vi "Device VI 1.4.vi"() -> ()   [LabVIEW 2017]
uses:
  <vilib>/Utility/error.llb/DialogType.ctl
  <vilib>/DAQmx/read.llb/DAQmx Read (Analog 1D Wfm NChan NSamp).vi
  <vilib>/DAQmx/create/channels.llb/DAQmx Create Channel (AI-Force-Bridge-Two-Point-Linear).vi
  <vilib>/DAQmx/configure/timing.llb/DAQmx Timing (Sample Clock).vi
  <vilib>/DAQmx/configure/trigger.llb/DAQmx Start Trigger (Digital Edge).vi
  <vilib>/DAQmx/configure/trigger.llb/DAQmx Start Trigger (Analog Edge).vi
  <vilib>/DAQmx/miscellaneous.llb/DAQmx Fill In Error Info.vi
  <resource>/objmgr/daqmx.rc
panel:
  in  "Pause":bool
  in  "Start":bool
  in  "Stop 3":bool
  in  "Spreadsheet Location":path=path "C:/Users/Julio/Desktop/Device Data/Test 2.xlsx" caption="Filename"
  in  "Units (Force)":i32(ring)=15875 items=["Newtons"=15875, "Pounds"=15876, "kgf"=15877, "From Custom Scale"=10065]
  in  "Physical Channel":tag="cDAQ2Mod1/ai0:1"
  in  "Sample Rate (Hz)":dbl=100.0
  in  "Samples per Loop":i32=100
  in  "scaling information":T1={"first electrical value"=0.0, "second electrical value"=2.0, "electrical units"=15897, "first physical value"=0.0, "second physical value"=100.0, "physical units"=15876} {"physical units" items=["Newtons"=15875, "Pounds"=15876, "kgf"=15877]; "electrical units" items=["Volts/Volt"=15896, "mVolts/Volt"=15897]}
  in  "Maximum Force":dbl=100.0
  in  "Minimum Force":dbl=-100.0
  in  "Trigger Type":T2(tab)
  in  "Digital Start Trigger Edge":i32(ring)=10280 caption="Edge" items=["Rising"=10280, "Falling"=10171]
  in  "Digital Start Trigger Source":tag="OnboardClock" caption="Source"
  in  "Digital Pause Trigger Pause When":i32(ring)=10192 caption="Pause When" items=["High"=10192, "Low"=10214]
  in  "Digital Pause Trigger Source":tag="/Dev1/PFI0" caption="Source"
  in  "Analog Start Trigger Level":dbl caption="Level" format="%0.2f"
  in  "Analog Start Trigger Hysteresis":dbl caption="Hysteresis" format="%.2f"
  in  "Analog Start Trigger Slope":i32(ring)=10280 caption="Slope" items=["Rising"=10280, "Falling"=10171]
  in  "Analog Start Trigger Source":string="APFI0" caption="Source"
  in  "Analog Pause Trigger Source":string="APFI0" caption="Source"
  in  "Analog Pause Trigger Pause When":i32(ring)=10093 caption="Pause When" items=["Above Level"=10093, "Below Level"=10107]
  in  "Analog Pause Trigger Level":dbl caption="Level" format="%.2f"
  in  "Bridge Information":T3={"Bridge Configuration"=10182, "Excitation Source"=10200, "Excitation Value"=2.5, "Nominal Resistance"=350.0} {"Excitation Source" items=["Internal"=10200, "External"=10167, "None"=10230]; "Bridge Configuration" items=["Full Bridge"=10182, "Half Bridge"=10187, "Quarter Bridge"=10270, "No Bridge"=10228]}
  out "Waveform Chart":waveform(dbl)[](graph)=[{"t0"=timestamp(3612864703.636625 s since 1904-01-01), "dt"=0.01, "Y"=[-0.0008285458908220164, -0.0008285458908220164, -0.0008285458908220164, -0.0008285458908220164, -0.0008285458908220164, -0.0008285458908220164, -0.0008285458908220164, -0.0008285458908220164, -0.0008285458908220164, -0.0008285458908220164, -0.0008285458908220164, -0.0008285458908220164, -0.0008285458908220164, -0.0008285458908220164, -0.0008285458908220164, -0.0008285458908220164, -0.0008285458908220164, -0.0008285458908220164, -0.0008285458908220164, -0.0008285458908220164, -0.0008285458908220164, -0.0008285458908220164, -0.0008285458908220164, -0.0008285458908220164, -0.0008285458908220164, -0.0008285458908220164, -0.0008285458908220164, -0.0008285458908220164, -0.0008285458908220164, -0.0008285458908220164, -0.0008285458908220164, -0.0008285458908220164, -0.0008285458908220164, -0.0008285458908220164, -0.0008285458908220164, -0.0008285458908220164, -0.0008285458908220164, -0.0008285458908220164, -0.0008285458908220164, -0.0008285458908220164, -0.0008285458908220164, -0.0008285458908220164, -0.0008285458908220164, -0.0008285458908220164, -0.0008285458908220164, -0.0008285458908220164, -0.0008285458908220164, -0.0008285458908220164, -0.0008285458908220164, -0.0008285458908220164, -0.0008285458908220164, -0.0008285458908220164, -0.0008285458908220164, -0.0008285458908220164, -0.0008285458908220164, -0.0008285458908220164, -0.0008285458908220164, -0.0008285458908220164, -0.0008285458908220164, -0.0008285458908220164, -0.0008285458908220164, -0.0008285458908220164, -0.0008285458908220164, -0.0008285458908220164, -0.0008285458908220164, -0.0008285458908220164, -0.0008285458908220164, -0.0008285458908220164, -0.0008285458908220164, -0.0008285458908220164, -0.0008285458908220164, -0.0008285458908220164, -0.0008285458908220164, -0.0008285458908220164, -0.0008285458908220164, -0.0008285458908220164, -0.0008285458908220164, -0.0008285458908220164, -0.0008285458908220164, -0.0008285458908220164, -0.0008285458908220164, -0.0008285458908220164, -0.0008285458908220164, -0.0008285458908220164, -0.0008285458908220164, -0.0008285458908220164, -0.0008285458908220164, -0.0008285458908220164, -0.0008285458908220164, -0.0008285458908220164, -0.0008285458908220164, -0.0008285458908220164, -0.0008285458908220164, -0.0008285458908220164, -0.0008285458908220164, -0.0008285458908220164, -0.0008285458908220164, -0.0008285458908220164, -0.0008285458908220164, -0.0008285458908220164], "attributes"=variant("NI_ChannelName"=variant(string "cDAQ2Mod1/ai0"), "NI_UnitDescription"=variant(string "Newtons"))}, {"t0"=timestamp(3612864703.636625 s since 1904-01-01), "dt"=0.01, "Y"=[0.006835503599282382, 0.006835503599282382, 0.006835503599282382, 0.006835503599282382, 0.006835503599282382, 0.006835503599282382, 0.006835503599282382, 0.006835503599282382, 0.006835503599282382, 0.006835503599282382, 0.006835503599282382, 0.006835503599282382, 0.006835503599282382, 0.006835503599282382, 0.006835503599282382, 0.006835503599282382, 0.006835503599282382, 0.006835503599282382, 0.006835503599282382, 0.006835503599282382, 0.006835503599282382, 0.006835503599282382, 0.006835503599282382, 0.006835503599282382, 0.006835503599282382, 0.006835503599282382, 0.006835503599282382, 0.006835503599282382, 0.006835503599282382, 0.006835503599282382, 0.006835503599282382, 0.006835503599282382, 0.006835503599282382, 0.006835503599282382, 0.006835503599282382, 0.006835503599282382, 0.006835503599282382, 0.006835503599282382, 0.006835503599282382, 0.006835503599282382, 0.006835503599282382, 0.006835503599282382, 0.006835503599282382, 0.006835503599282382, 0.006835503599282382, 0.006835503599282382, 0.006835503599282382, 0.006835503599282382, 0.006835503599282382, 0.006835503599282382, 0.008906868326337657, 0.008906868326337657, 0.008906868326337657, 0.008906868326337657, 0.008906868326337657, 0.008906868326337657, 0.008906868326337657, 0.008906868326337657, 0.008906868326337657, 0.008906868326337657, 0.008906868326337657, 0.008906868326337657, 0.008906868326337657, 0.008906868326337657, 0.008906868326337657, 0.008906868326337657, 0.008906868326337657, 0.008906868326337657, 0.008906868326337657, 0.008906868326337657, 0.008906868326337657, 0.008906868326337657, 0.008906868326337657, 0.008906868326337657, 0.008906868326337657, 0.008906868326337657, 0.008906868326337657, 0.008906868326337657, 0.008906868326337657, 0.008906868326337657, 0.008906868326337657, 0.008906868326337657, 0.008906868326337657, 0.008906868326337657, 0.008906868326337657, 0.008906868326337657, 0.008906868326337657, 0.008906868326337657, 0.008906868326337657, 0.008906868326337657, 0.008906868326337657, 0.008906868326337657, 0.008906868326337657, 0.008906868326337657, 0.008906868326337657, 0.008906868326337657, 0.008906868326337657, 0.008906868326337657, 0.008906868326337657, 0.008906868326337657], "attributes"=variant("NI_ChannelName"=variant(string "cDAQ2Mod1/ai1"), "NI_UnitDescription"=variant(string "Newtons"))}]
  # "Settings"
  # "This trigger type is not supported in continuous sample timing. \n\nRefer to your device documentation for more information on which triggers are supported."
  # "This trigger type is not supported in continuous sample timing. \n\nRefer to your device documentation for more information on which triggers are supported."
  # "Data"
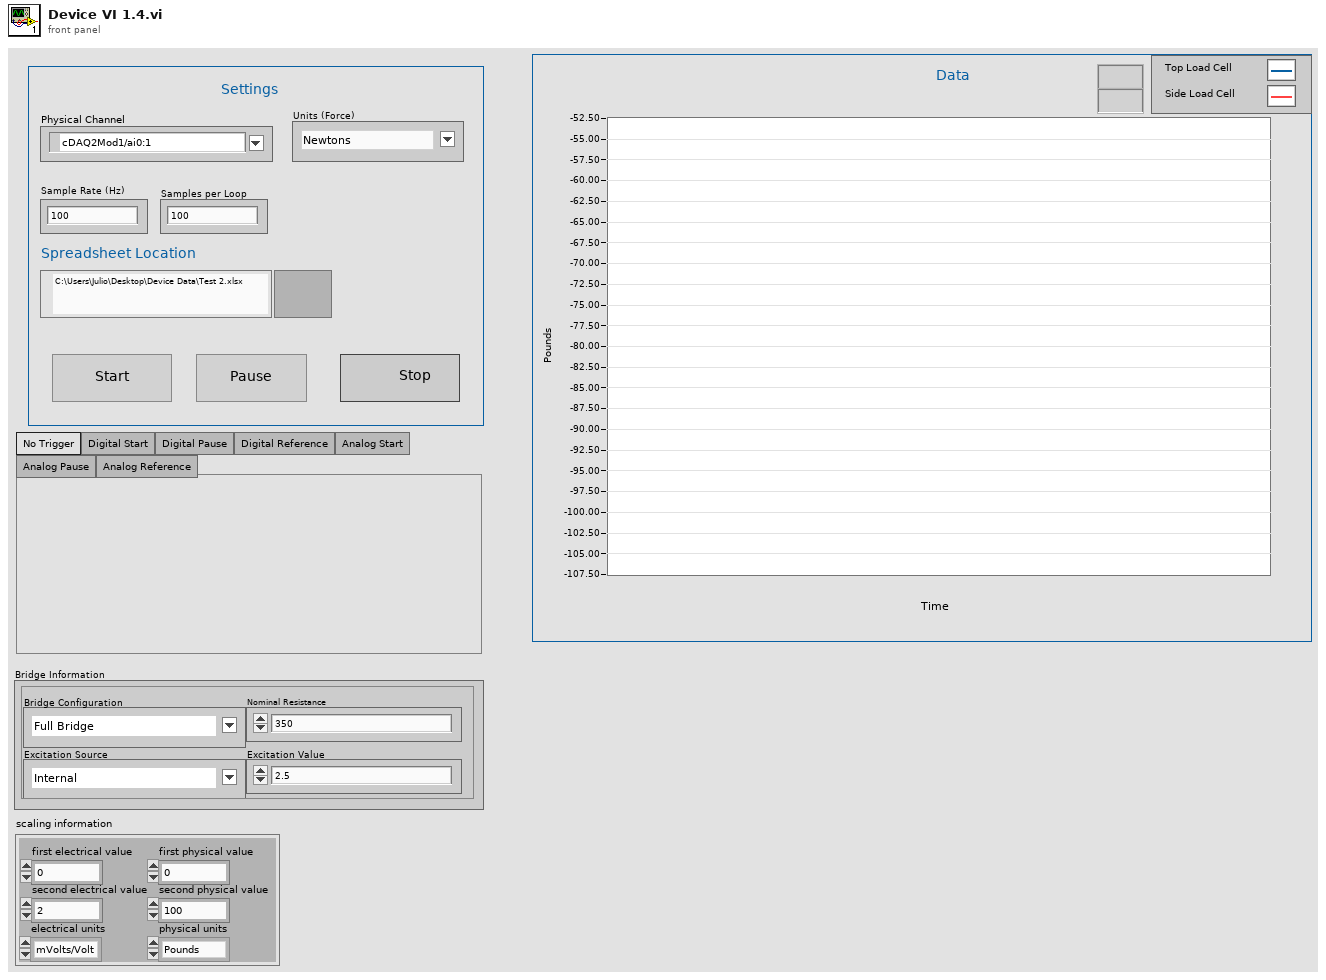
[diagram p1: front panel]
types:
  T1 = cluster{"first electrical value":dbl, "second electrical value":dbl, "electrical units":i32, "first physical value":dbl, "second physical value":dbl, "physical units":i32}
  T2 = enum32{"No Trigger", "Digital Start", "Digital Pause", "Digital Reference", "Analog Start", "Analog Pause", "Analog Reference"}
  T3 = cluster{"Bridge Configuration":i32, "Excitation Source":i32, "Excitation Value":dbl, "Nominal Resistance":dbl}
  T4 = typedef "DialogType.ctl" = u16
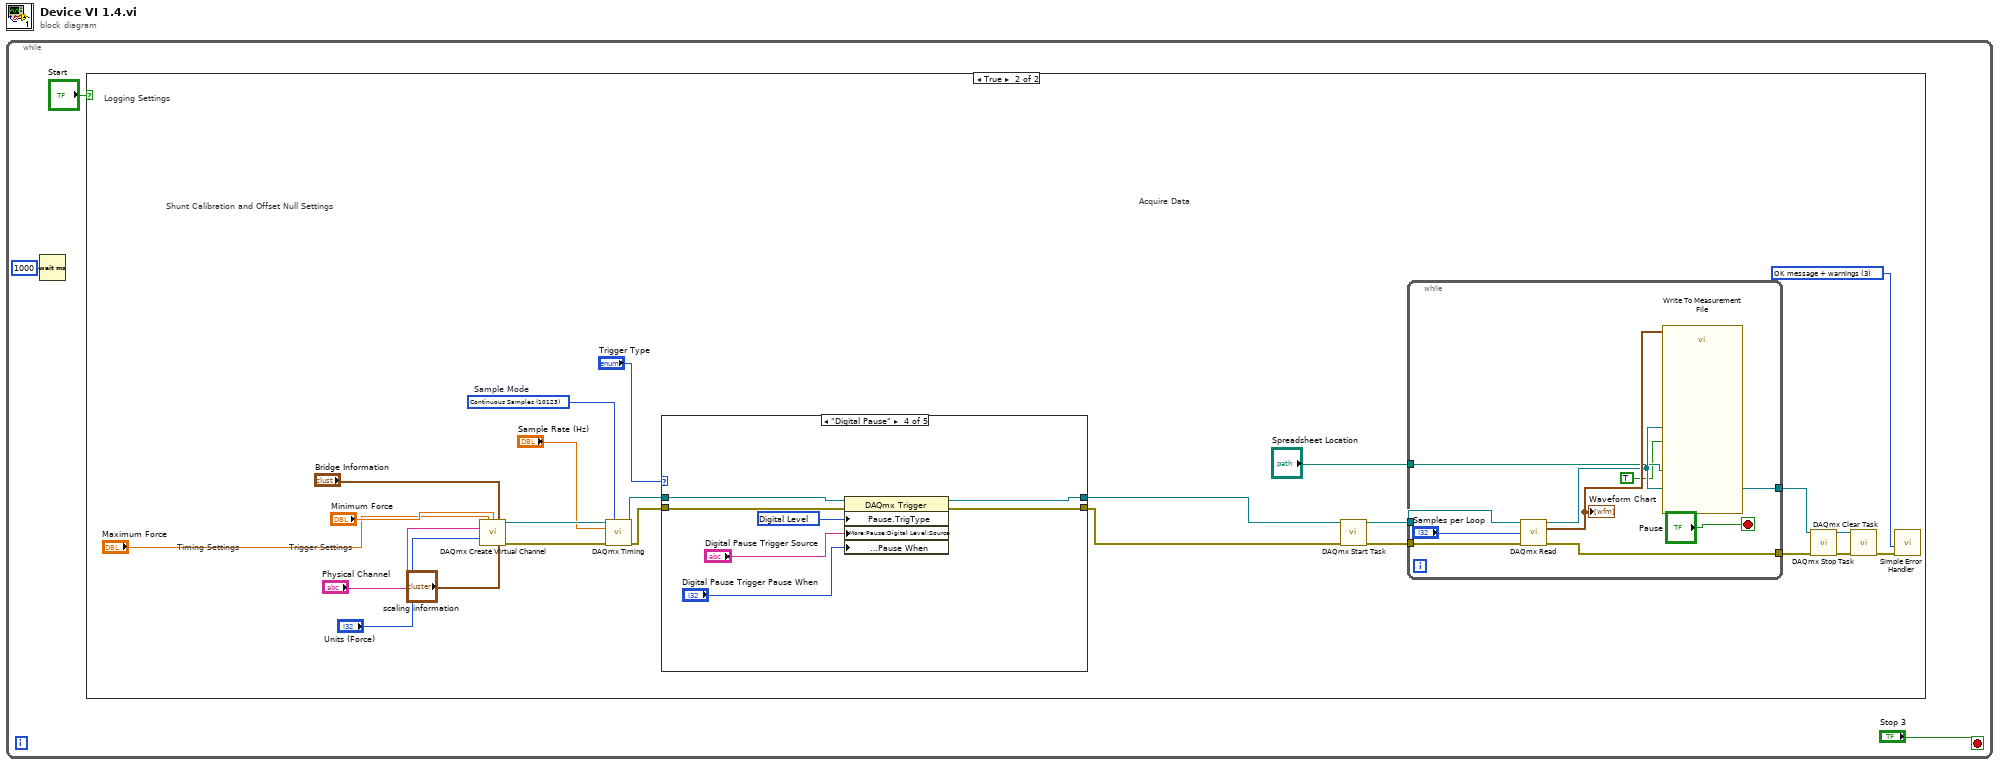
[diagram p0: block diagram]
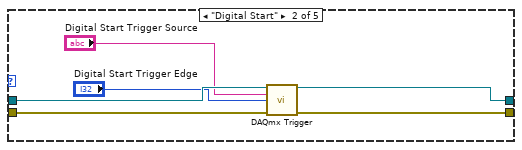
[diagram p4: hidden frame]
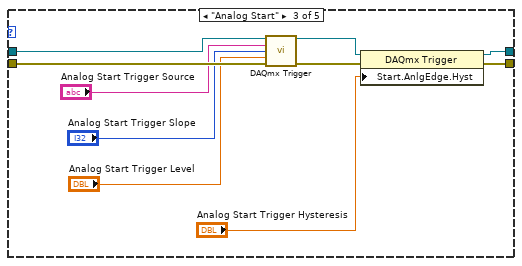
[diagram p5: hidden frame]
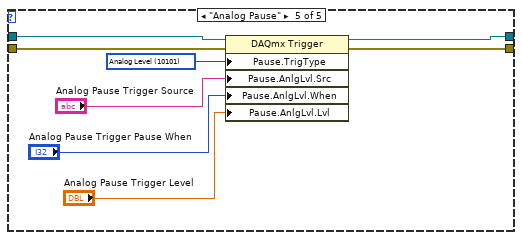
[diagram p6: hidden frame]
diagram:
  n1 = while {
    stop <- "Stop 3" stop-if-true
    n2 = Wait (ms)(milliseconds to wait=u32 1000) -> ()  [unwired: 1 out]
    n3 = case shown="True" "Start" {
      frame False {
      }
      frame True {
        w14 = T4 3 items=["no dialog", "OK message", "continue or stop message", "OK message + warnings", "continue/stop + warnings"] ("type of dialog (OK msg:1)")
        w27 = 10123 items=["Finite Samples"=10178, "Continuous Samples"=10123, "Hardware Timed Single Point"=12522]  # Sample Mode
        # "Trigger Settings"
        # "Logging Settings"
        # "Acquire Data"
        # "Shunt Calibration and Offset Null Settings"
        # "Timing Settings"
        n4 = call-poly <vilib>:"DAQmx Create Virtual Channel.vi"("maximum value"="Maximum Force", "minimum value"="Minimum Force", "bridge information"="Bridge Information", "physical channels"="Physical Channel", "units"="Units (Force)", "scaling information"="scaling information") -> ("task out"=w25:refnum<k21>, "error out"=w26:errorcluster)  [unwired: 8 in]
        n5 = call-poly <vilib>:"DAQmx Timing.vi"("task/channels in"=w25, "sample mode"=w27, "rate"="Sample Rate (Hz)", "error in"=w26) -> ("task out"=w9:refnum<k21>, "error out"=w8:errorcluster)  [unwired: 10 in]
        n6 = case shown="\"Digital Pause\"" "Trigger Type" {
          tunnel: w9 -> [w29 w35 w45 w52 w60]
          tunnel: w8 -> [w28 w34 w44 w49 w57]
          tunnel: [w29 w33 w42 w51 w59] -> w6
          tunnel: [w28 w32 w41 w50 w58] -> w5
          frame "No Trigger", Default {
          }
          frame "Digital Start" {
            n7 = call-poly <vilib>:"DAQmx Trigger.vi"("task/channels in"=w35, "source"="Digital Start Trigger Source", "edge"="Digital Start Trigger Edge", "error in"=w34) -> ("task out"=w33:refnum<k21>, "error out"=w32:errorcluster)  [unwired: 10 in]
          }
          frame "Analog Start" {
            n8 = call-poly <vilib>:"DAQmx Trigger.vi"("task/channels in"=w45, "source"="Analog Start Trigger Source", "slope"="Analog Start Trigger Slope", "level"="Analog Start Trigger Level", "error in"=w44) -> ("task out"=w40:refnum<k21>, "error out"=w39:errorcluster)  [unwired: 9 in]
            n9 = property class="DAQmx Trigger"(reference=w40, error in=w39, "Start.AnlgEdge.Hyst"="Analog Start Trigger Hysteresis") -> (reference out=w42:refnum<k21>, error out=w41:errorcluster)
          }
          frame "Digital Pause" {
            w48 = 10152 items=["Analog Level"=10101, "Analog Window"=10103, "Digital Level"=10152, "Digital Pattern"=10398, "None"=10230] ("Pause.TrigType")
            n10 = property class="DAQmx Trigger"(reference=w52, error in=w49, "Pause.TrigType"=w48, "More:Pause:Digital Level:Source"="Digital Pause Trigger Source", "More:Pause:Digital Level:Pause When"="Digital Pause Trigger Pause When") -> (reference out=w51:refnum<k21>, error out=w50:errorcluster)
          }
          frame "Analog Pause" {
            w56 = 10101 items=["Analog Level"=10101, "Analog Window"=10103, "Digital Level"=10152, "Digital Pattern"=10398, "None"=10230] ("Pause.TrigType")
            n11 = property class="DAQmx Trigger"(reference=w60, error in=w57, "Pause.TrigType"=w56, "Pause.AnlgLvl.Src"="Analog Pause Trigger Source", "Pause.AnlgLvl.When"="Analog Pause Trigger Pause When", "Pause.AnlgLvl.Lvl"="Analog Pause Trigger Level") -> (reference out=w59:refnum<k21>, error out=w58:errorcluster)
          }
        }
        n12 = call <vilib>:"DAQmx Start Task.vi"("task/channels in"=w6, "error in"=w5) -> ("task out"=w24:refnum<k21>, "error out"=w23:errorcluster)  [unwired: 12 in]
        n13 = while {
          tunnel: w24 -> [w69]
          tunnel: w23 -> [w68]
          tunnel: [w67] -> w17
          tunnel: [w64] -> w18
          tunnel: "Spreadsheet Location" -> [w63]
          stop <- "Pause" stop-if-true
          n14 = call-poly <vilib>:"DAQmx Read.vi"("task/channels in"=w69, "number of samples per channel"="Samples per Loop", "error in"=w68) -> ("task out"=w64:refnum<k21>, "data"=w65:waveform(dbl)[], "error out"=w67:errorcluster)  [unwired: 10 in]
          "Waveform Chart" <- w65
          n15 = call "Write To Measurement File"("Signals"=w65, "Enable"=TRUE ("Append"), "Filename"=w63, "DAQmx Task"=w64) -> ()  [unwired: 13 in, 3 out]
        }
        n16 = call <vilib>:"DAQmx Stop Task.vi"("task/channels in"=w18, "error in"=w17) -> ("task out"=w16:refnum<k21>, "error out"=w15:errorcluster)  [unwired: 12 in]
        n17 = call <vilib>:"DAQmx Clear Task.vi"("task in"=w16, "error in"=w15) -> ("error out"=w22:errorcluster)  [unwired: 13 in]
        n18 = call <vilib>:"Simple Error Handler.vi"("type of dialog (OK msg:1)"=w14, "error in (no error)"=w22) -> ()  [unwired: 3 in, 5 out]
      }
    }
  }
